vi "Sandbox-Fpga-Caller.vi"() -> ()   [LabVIEW 2017]
uses:
  <vilib>/FPGAPlugInAG/PXIe-6592R/niLvFpga_Open_PXIe-6592R.vi
  <vilib>/rvi/interface/common/dynamic/niFpgaDynamicAddResources.vi
  <vilib>/Utility/error.llb/Error Cluster From Error Code.vi
  <vilib>/rvi/errors/niLvFpgaAdjustHostInterfaceError.vi
  <vilib>/FPGAPlugInAG/Dynamic/niLvFpga_Close_Dynamic.vi
  <vilib>/rvi/interface/nirviOpenFPGA/nirviOpenFPGA.xnode
  FPGA Bitfiles/0710GigabitCLIP_FPGATarget_Fpga-Feedback-Te_IzNnnJvoFyg.lvbitx
  <vilib>/rvi/interface/nirviMethod/nirviMethod.xnode
  <vilib>/rvi/interface/nirviCloseFPGA/nirviCloseFPGA.xnode
  <vilib>/FPGAPlugInAG/Dynamic/niLvFpga_ReadFifo_Dynamic.vi
  <vilib>/rvi/errors/niLvFpgaMergeErrorWithErrorCode.vi
panel:
  out "error out":errorcluster
  out "Data":u64[](array[numeric])=[18446744073709551615, 18446744073709551615, 0, 2, 18446744073709551615, 18446744073709551615, 3, 6, 18446744073709551615, 18446744073709551615, 7, 10, 18446744073709551615, 18446744073709551615, 11, 14, 18446744073709551615, 18446744073709551615, 15, 18] format="%.0x"
  in  "error in":errorcluster
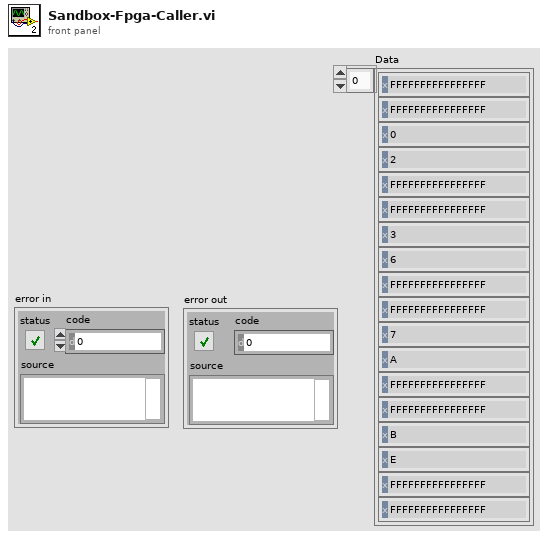
[diagram p1: front panel]
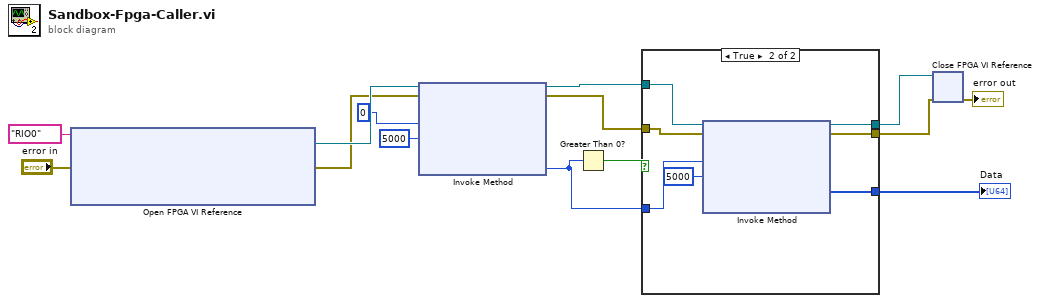
[diagram p0: block diagram]
diagram:
  n1 = xnode "Open FPGA VI Reference"("error in"="error in", "resource name"=tag "RIO0") -> ("FPGA VI Reference Out"=w13:refnum<k20>, "error out"=w12:errorcluster)
  n2 = xnode "Invoke Method"("FPGA VI Reference In"=w13, "error in"=w12, "Number of Elements"=u32 0, "Timeout (ms)"=5000) -> ("FPGA VI Reference Out"=w9:refnum<k20>, "error out"=w8:errorcluster, "Elements Remaining"=w7:u32)  [unwired: 1 out]
  n3 = Greater Than 0?(x=w7) -> (x > 0?=w6:bool)
  n4 = case shown="True" w6 {
    tunnel: w7 -> [_ w23]
    tunnel: w9 -> [w15 w21]
    tunnel: w8 -> [w16 w20]
    tunnel: [_ w19] -> w5
    tunnel: [w16 w18] -> w4
    tunnel: [w15 w17] -> w3
    frame False {
    }
    frame True {
      n5 = xnode "Invoke Method"("FPGA VI Reference In"=w21, "error in"=w20, "Number of Elements"=w23, "Timeout (ms)"=5000) -> ("FPGA VI Reference Out"=w17:refnum<k20>, "error out"=w18:errorcluster, "Data"=w19:u64[])  [unwired: 1 out]
    }
  }
  "Data" <- w5
  n6 = xnode "Close FPGA VI Reference"("FPGA VI Reference In"=w3, "error in"=w4) -> ("error out"=→"error out":errorcluster)
